vi "FRCts20_WebMethods_Globals.vi"() -> ()   [LabVIEW 2014, in "FRCts20_WebMethods.lvlib"]
uses:
  FRCts20_WebMethods.lvlib
panel:
  in  "Esp Script Path":string="/static/esp/scripts/FRCts20_Support.esp"
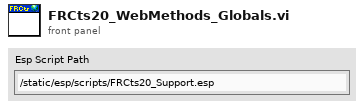
[diagram p1: front panel]
diagram:
